vi "worksheet fit to pages.vi"(8 "error in (no error)":errorcluster, 9 "height":u16, 10 "width":u16, 11 "worksheet":u32) -> (0 "error out":errorcluster)   [LabVIEW 2015, in "xlsxwriter.lvlib"]
doc: "void worksheet_fit_to_pages(lxw_worksheet worksheet, uint16_t width, uint16_t height);"
uses:
  xlsxwriter.lvlib
  xlsxwriter.dll
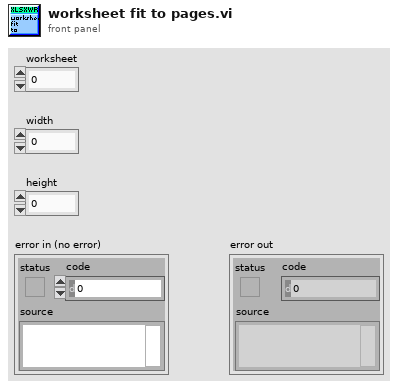
[diagram p1: front panel]
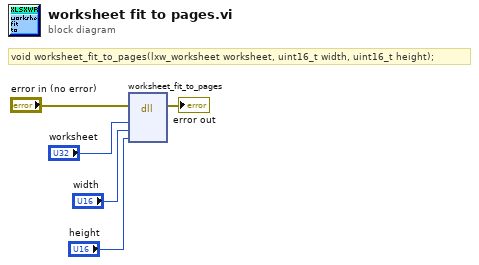
[diagram p0: block diagram]
diagram:
  # "void worksheet_fit_to_pages(lxw_worksheet worksheet, uint16_t width, uint16_t height);"
  n1 = dll-call lib="C:/Users/WDAGUtilityAccount/Desktop/lv_vis_added_cell/xlsxwriter.*" fn="worksheet_fit_to_pages"(error in="error in (no error)", "worksheet"="worksheet", "width"="width", "height"="height") -> (error out=→"error out":errorcluster)  [unwired: 6 in, 1 out]
